vi "T7 Cal Constants Tool.vi"() -> (0 "error out":errorcluster)   [LabVIEW 2020]
uses:
  <vilib>/Utility/file.llb/Read From Spreadsheet File (DBL).vi
  <vilib>/Utility/file.llb/Write To Spreadsheet File (DBL).vi
panel:
  in  "Flash Key":i32 format="%x"
  in  "Read Cluster from File":bool
  in  "Write Cluster to File":bool
  in  "Cluster":T1
  out "Array":dbl[](array[numeric])
  out "# Reads":i32
  in  "Read Cal":bool
  in  "Exit":bool
  out "# Writes":i32
  in  "Write Cal":bool
  out "Error String":string="No Error"
  out "ConnectionType Out":i32
  out "DeviceType Out":i32
  in  "Identifier":string="LJM_idANY"
  in  "ConnectionType":string="LJM_ctANY"
  in  "DeviceType":string="LJM_dtANY"
  # "When you click \"Read\" or \"Write\", this program does open-write-read-close."
  # "0xA7863777 is the key\nto write cal constants.\n\nPower-cycle might be required for\nnew constants to take effect."
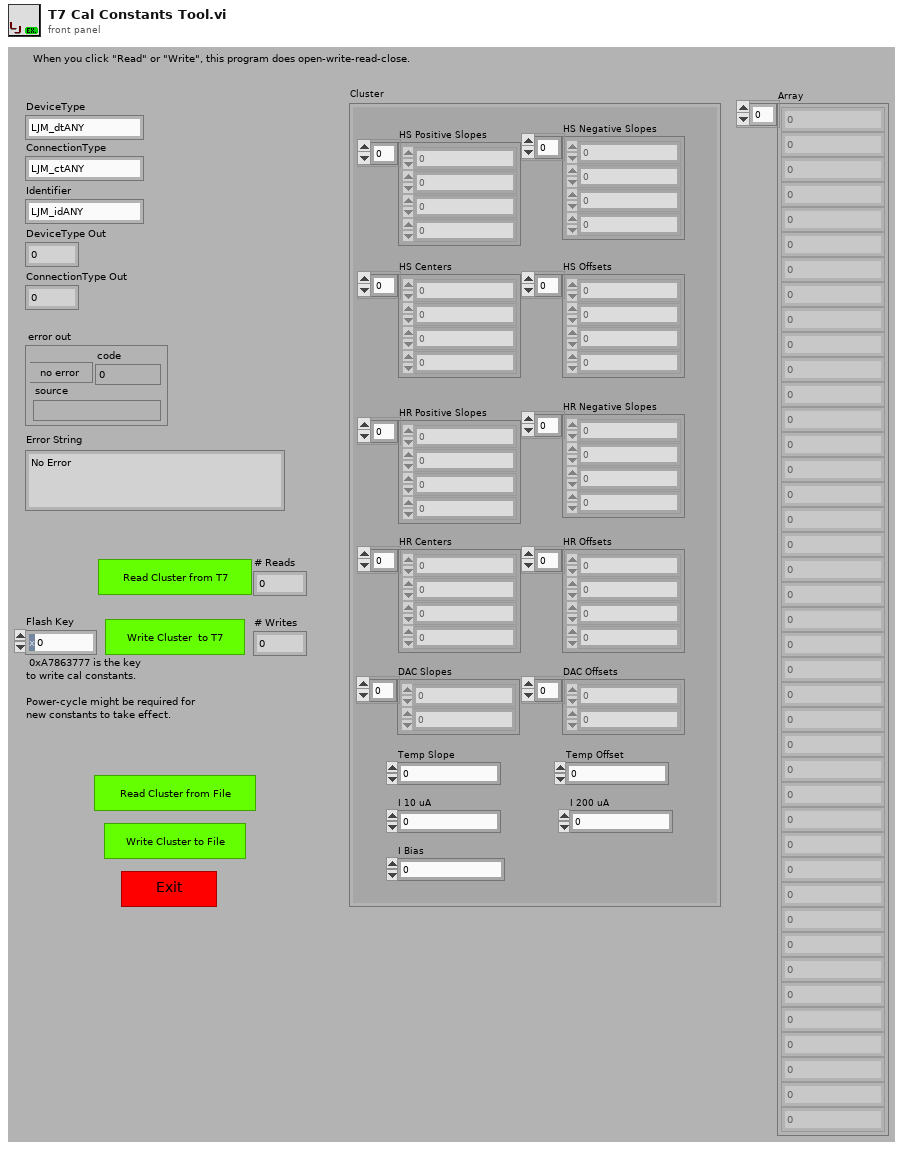
[diagram p1: front panel]
types:
  T1 = cluster{"HS Positive Slopes":dbl[], "HS Negative Slopes":dbl[], "HS Centers":dbl[], "HS Offsets":dbl[], "HR Positive Slopes":dbl[], "HR Negative Slopes":dbl[], "HR Centers":dbl[], "HR Offsets":dbl[], "DAC Slopes":dbl[], "DAC Offsets":dbl[], "Temp Slope":dbl, "Temp Offset":dbl, "I 10 uA":dbl, "I 200 uA":dbl, "I Bias":dbl}
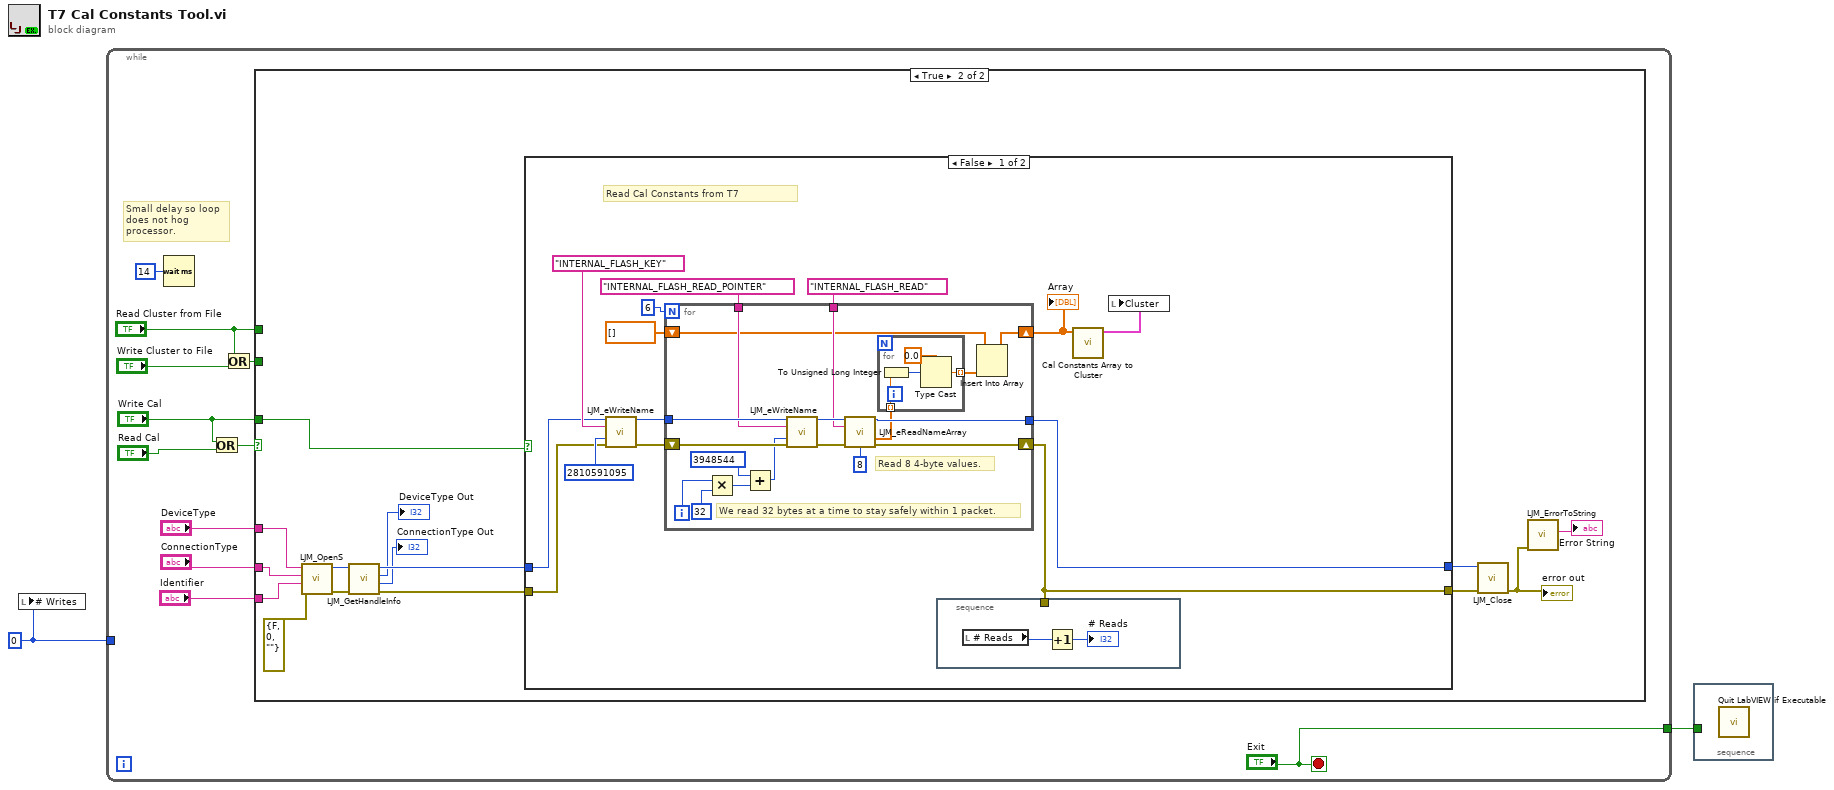
[diagram p0: block diagram]
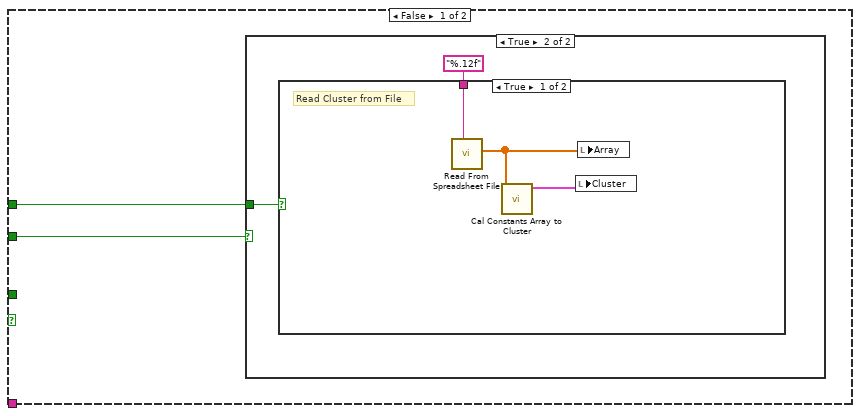
[diagram p2: hidden frame]
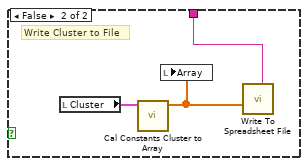
[diagram p4: hidden frame]
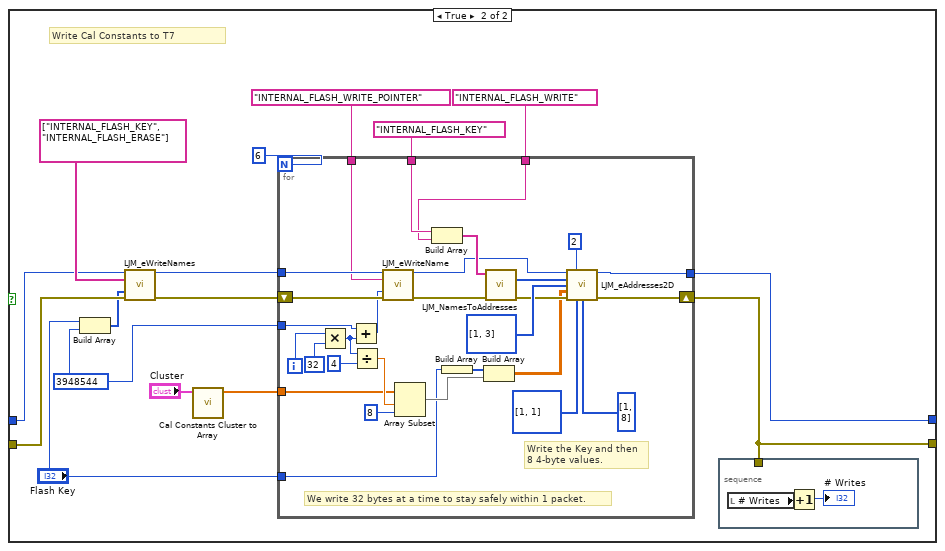
[diagram p5: hidden frame]
diagram:
  w1 = 0 ("# Writes")
  n1 = local write "# Writes"(w1) -> ()
  n2 = while {
    tunnel: w1 -> [_]
    tunnel: ["Exit"] -> w2
    stop <- "Exit" stop-if-true
    # "Small delay so loop\ndoes not hog\nprocessor."
    n3 = Wait (ms)(milliseconds to wait=u32 14) -> ()  [unwired: 1 out]
    n4 = Or(x="Write Cal", y="Read Cal") -> (x .or. y?=w8:bool)
    n5 = Or(x="Read Cluster from File", y="Write Cluster to File") -> (x .or. y?=w4:bool)
    n6 = case shown="True" w8 {
      tunnel: "Identifier" -> [_ w28]
      tunnel: "ConnectionType" -> [_ w27]
      tunnel: "DeviceType" -> [_ w26]
      tunnel: "Write Cal" -> [_ w24]
      tunnel: w4 -> [w15 _]
      tunnel: "Read Cluster from File" -> [w14 _]
      frame False {
        n7 = case shown="True" w15 {
          tunnel: w14 -> [_ w17]
          frame False {
          }
          frame True {
            n8 = case shown="True" w17 {
              tunnel: "%.12f" ("format (%.3f)") -> [w18 w21]
              frame True {
                # "Read Cluster from File"
                n9 = call-poly <vilib>:"Read From Spreadsheet File.vi"("format (%.3f)"=w18) -> ("first row"=w20:dbl[])  [unwired: 6 in, 4 out]
                n10 = call "Cal Constants Array to Cluster.vi"("Array"=w20) -> ("Cluster"=w19:T1)  [unwired: 10 in]
                n11 = local write "Cluster"(w19) -> ()
                n12 = local write "Array"(w20) -> ()
              }
              frame False {
                # "Write Cluster to File"
                n13 = local read "Cluster"() -> (w23:T1)
                n14 = call "Cal Constants Cluster to Array.vi"("Cluster"=w23) -> ("Array"=w22:dbl[])  [unwired: 10 in]
                n15 = local write "Array"(w22) -> ()
                n16 = call-poly <vilib>:"Write To Spreadsheet File.vi"("format (%.3f)"=w21, "1D data"=w22) -> ()  [unwired: 6 in, 1 out]
              }
            }
          }
        }
      }
      frame True {
        n17 = call "LJM_OpenS.vi"("error in"=errorcluster {"status"=FALSE, "code"=0, "source"=""} ("error in (no error)"), "Identifier"=w28, "ConnectionType"=w27, "DeviceType"=w26) -> ("error out"=w37:errorcluster, "Handle"=w35:i32)  [unwired: 6 in]
        n18 = call "LJM_GetHandleInfo.vi"("error in"=w37, "Handle In"=w35) -> ("error out"=w36:errorcluster, "ConnectionType"=→"ConnectionType Out":i32, "DeviceType"=→"DeviceType Out":i32, "Handle Out"=w34:i32)  [unwired: 2 in, 4 out]
        n19 = case shown="False" w24 {
          tunnel: w36 -> [w44 w84]
          tunnel: w34 -> [w45 w83]
          tunnel: [w43 w89] -> w33
          tunnel: [w42 w88] -> w25
          frame False {
            # "Read Cal Constants from T7"
            n20 = call "LJM_eWriteName.vi"("Handle In"=w45, "Name"="INTERNAL_FLASH_KEY" ("String"), "Value"=u32 2810591095 ("NumFrames"), "error in"=w44) -> ("Handle Out"=w48:i32, "error out"=w47:errorcluster)  [unwired: 10 in]
            n21 = for {
              N: 6 -> [_]
              tunnel: w48 -> [w68]
              tunnel: [w55] -> w43
              shift-right: [w70] -> w42
              shift-left: w47 -> [w69]
              tunnel: "INTERNAL_FLASH_READ" ("Name") -> [w65]
              tunnel: "INTERNAL_FLASH_READ_POINTER" ("String") -> [w64]
              shift-right: [w58] -> w41
              shift-left: sgl[] [] -> [w57]
              i -> [w63]
              # "We read 32 bytes at a time to stay safely within 1 packet."
              # "Read 8 4-byte values."
              n22 = Multiply(x=w63, y=32 ("NumValues")) -> (x*y=w60:i32)
              n23 = Add(x=u32 3948544 ("NumFrames"), y=w60) -> (x+y=w59:u32)
              n24 = call "LJM_eWriteName.vi"("Handle In"=w68, "Name"=w64, "Value"=w59, "error in"=w69) -> ("Handle Out"=w67:i32, "error out"=w66:errorcluster)  [unwired: 10 in]
              n25 = call "LJM_eReadNameArray.vi"("Handle In"=w67, "Name"=w65, "error in"=w66, "NumValues"=8) -> ("Handle Out"=w55:i32, "aValues"=w54:dbl[], "error out"=w70:errorcluster)  [unwired: 8 in, 1 out]
              n26 = for {
                tunnel: [w74] -> w56 mode=indexing
                tunnel: w54 -> [w71] mode=indexing
                n27 = To Unsigned Long Integer(number=w71) -> (unsigned 32bit integer=w73:u32)
                n28 = Type Cast(type=sgl 0.0, x=w73) -> (*(type *) &x=w74:sgl)
              }
              n29 = Insert Into Array(array=w57, new element=w56) -> (w58:sgl[])  [unwired: 1 in]
            }
            "Array" <- w41
            n30 = stacked-sequence {
              tunnel: w42 -> [_]
              frame #0 {
                n31 = local read "# Reads"() -> (w75:i32)
                n32 = Increment(x=w75) -> (x+1=→"# Reads":i32)
              }
            }
            n33 = call "Cal Constants Array to Cluster.vi"("Array"=w41) -> ("Cluster"=w40:T1)  [unwired: 10 in]
            n34 = local write "Cluster"(w40) -> ()
          }
          frame True {
            w79 = u32 3948544 ("NumFrames")
            # "Write Cal Constants to T7"
            n35 = Build Array("Flash Key", w79) -> (w80:u32[])
            n36 = call "LJM_eWriteNames.vi"("Handle In"=w83, "aNames"=string[] ["INTERNAL_FLASH_KEY", "INTERNAL_FLASH_ERASE"], "aValuesIn"=w80, "error in"=w84) -> ("Handle Out"=w82:i32, "error out"=w81:errorcluster)  [unwired: 9 in, 1 out]
            n37 = call "Cal Constants Cluster to Array.vi"("Cluster"="Cluster") -> ("Array"=w77:dbl[])  [unwired: 10 in]
            n38 = for {
              N: 6 -> [_]
              tunnel: w82 -> [w122]
              tunnel: [w110] -> w89
              shift-right: [w111] -> w88
              shift-left: w81 -> [w123]
              tunnel: "INTERNAL_FLASH_WRITE" ("Name") -> [w103]
              tunnel: "INTERNAL_FLASH_WRITE_POINTER" ("String") -> [w121]
              tunnel: w79 -> [w118]
              tunnel: w77 -> [w113]
              tunnel: "INTERNAL_FLASH_KEY" ("String") -> [w104]
              tunnel: "Flash Key" -> [w96]
              i -> [w120]
              w98 = i32[] [1, 1] items=["Read", "Write"] ("aWrites")
              # "Write the Key and then\n8 4-byte values."
              # "We write 32 bytes at a time to stay safely within 1 packet."
              n39 = Multiply(x=w120, y=32 ("NumValues")) -> (x*y=w116:i32)
              n40 = Add(x=w118, y=w116) -> (x+y=w119:u32)
              n41 = Divide(x=w116, y=4) -> (x/y=w114:dbl)
              n42 = call "LJM_eWriteName.vi"("Handle In"=w122, "Name"=w121, "Value"=w119, "error in"=w123) -> ("Handle Out"=w101:i32, "error out"=w106:errorcluster)  [unwired: 10 in]
              n43 = Array Subset(array=w113, index=w114, length=8) -> (w109:dbl[])
              n44 = Build Array(w104, w103) -> (w102:string[])
              n45 = Build Array(w96) -> (w108:i32[])
              n46 = Build Array(w108, w109) -> (w95:dbl[][])
              n47 = call "LJM_NamesToAddresses.vi"("error in"=w106, "aNames"=w102) -> ("error out"=w105:errorcluster, "aAddresses"=w100:i32[])  [unwired: 7 in, 1 out]
              n48 = call "LJM_eAddresses2D.vi"("Handle In"=w101, "NumFrames (Auto-Detect)"=2, "aAddresses"=w100, "aTypes"=i32[] [1, 3], "aValuesIn"=w95, "error in"=w105, "aWrites"=w98, "aNumValues"=i32[] [1, 8]) -> ("Handle Out"=w110:i32, "error out"=w111:errorcluster)  [unwired: 4 in, 2 out]
            }
            n49 = stacked-sequence {
              tunnel: w88 -> [_]
              frame #0 {
                n50 = local read "# Writes"() -> (w94:i32)
                n51 = Increment(x=w94) -> (x+1=→"# Writes":i32)
              }
            }
          }
        }
        n52 = call "LJM_Close.vi"("error in"=w25, "Handle"=w33) -> ("error out"=w30:errorcluster)  [unwired: 9 in]
        "error out" <- w30
        n53 = call "LJM_ErrorToString.vi"("error in"=w30) -> ("String"=→"Error String":string)  [unwired: 10 in]
      }
    }
  }
  n54 = stacked-sequence {
    tunnel: w2 -> [_]
    frame #0 {
      n55 = call "Quit LabVIEW if Executable.vi"() -> ()  [unwired: 1 in]
    }
  }
